vi "Auton-MoveVector.vi"(9 "Angle":dbl, 10 "Distance":dbl) -> (2 "Done?":bool)   [LabVIEW 2014]
uses:
  Vector.ctl
  Robot Global Data.vi
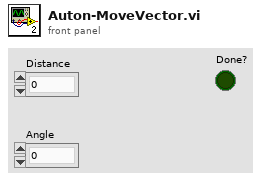
[diagram p1: front panel]
types:
  T1 = typedef "Vector.ctl" = cluster{"Magnitude":dbl, "Angle":dbl}
  T2 = typedef "WPI_EncoderDevRef.ctl" = cluster{"DevStatus":errorcluster, "EncoderIndex":T3, "CounterIndex":T4, "DistancePerCount":dbl, "Decoding Type":T5}
  T3 = typedef "FPGA_EncoderIdx.ctl" = enum8{"Enc 0", "Enc 1", "Enc 2", "Enc 3", "Enc 4", "Enc 5", "Enc 6", "Enc 7", "Invalid"}
  T4 = typedef "FPGA_CounterCtrSystemIndex.ctl" = enum8{"Ctr 0", "Ctr 1", "Ctr 2", "Ctr 3", "Ctr 4", "Ctr 5", "Ctr 6", "Ctr 7", "Invalid"}
  T5 = typedef "WPI_EncoderType.ctl" = enum16{"1x", "2x", "4x"}
  T6 = typedef "WPI_GyroDevRef.ctl" = cluster{"DevStatus":errorcluster, "Analog Module":T7, "Analog Channel":T8, "Offset":dbl, "Gain (VoltsPerDegree/Second)":dbl}
  T7 = typedef "FPGA_TypedefAnalogModule.ctl" = enum16{"Controller 1"}
  T8 = typedef "FPGA_AIChannel.ctl" = enum8{"AI 0", "AI 1", "AI 2", "AI 3", "AI MXP 0", "AI MXP 1", "AI MXP 2", "AI MXP 3", "Invalid"}
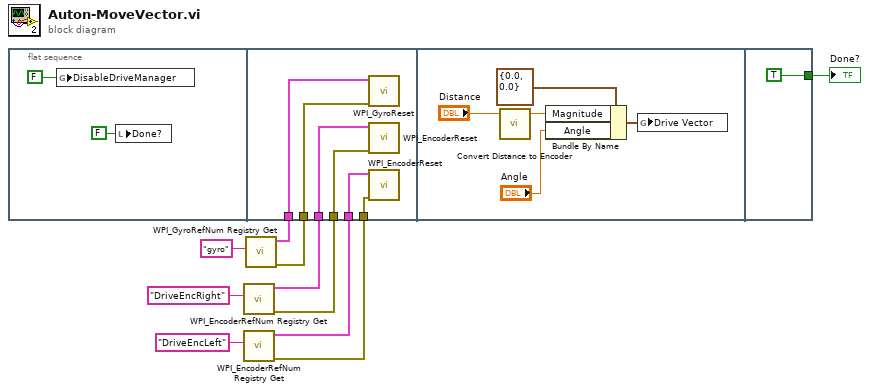
[diagram p0: block diagram]
diagram:
  n1 = flat-sequence {
    tunnel: w7 -> [w17]
    tunnel: w6 -> [w18]
    tunnel: w5 -> [w16]
    tunnel: w4 -> [w15]
    tunnel: w2 -> [w14]
    tunnel: w1 -> [w13]
    tunnel: [TRUE] -> w10
    frame #0 {
      n2 = global write "Robot Global Data.vi" "DisableDriveManager"(FALSE) -> ()
      n3 = local write "Done?"(FALSE ("Done?")) -> ()
    }
    frame #1 {
      n4 = call <vilib>:"WPI_GyroReset.vi"("error in (no error)"=w13, "GyroDevRef"=w14) -> ()  [unwired: 8 in, 2 out]
      n5 = call <vilib>:"WPI_EncoderReset.vi"("error in (no error)"=w16, "EncoderDevRef"=w15) -> ()  [unwired: 8 in, 2 out]
      n6 = call <vilib>:"WPI_EncoderReset.vi"("error in (no error)"=w18, "EncoderDevRef"=w17) -> ()  [unwired: 8 in, 2 out]
    }
    frame #2 {
      n7 = call "Convert Distance to Encoder.vi"("Dist (ft)"="Distance") -> ("Encoder"=w20:dbl)  [unwired: 4 in]
      n8 = Bundle By Name(cluster=T1 {"Magnitude"=0.0, "Angle"=0.0} ("Cluster"), "Magnitude"=w20, "Angle"="Angle") -> (w21:T1)
      n9 = global write "Robot Global Data.vi" "Drive Vector"(w21) -> ()
    }
    frame #3 {
    }
  }
  n10 = call <vilib>:"WPI_EncoderRefNum Registry Get.vi"("refnum name"="DriveEncRight") -> ("error out"=w5:errorcluster, "EncoderDevRef"=w4:T2)  [unwired: 9 in]
  n11 = call <vilib>:"WPI_EncoderRefNum Registry Get.vi"("refnum name"="DriveEncLeft") -> ("error out"=w6:errorcluster, "EncoderDevRef"=w7:T2)  [unwired: 9 in]
  n12 = call <vilib>:"WPI_GyroRefNum Registry Get.vi"("refnum name"="gyro") -> ("error out"=w1:errorcluster, "GyroDevRef"=w2:T6)  [unwired: 9 in]
  "Done?" <- w10
